vi "test Read Event.vi"(11 "Test Case In":refnum<class "Test PCANBasic.lvclass">) -> (0 "error out":errorcluster, 3 "Test Case Out":refnum<class "Test PCANBasic.lvclass">)   [LabVIEW 2020, in "Test PCANBasic.lvclass"]
uses:
  Test PCANBasic.lvclass
  Test PCANBasic.lvclass/Test PCANBasic.ctl
  C:/Program Files/National Instruments/LabVIEW 2026/vi.lib/Astemes/LUnit/Test Case.lvclass
  C:/Program Files/National Instruments/LabVIEW 2026/vi.lib/Astemes/LUnit/LUnit Runnable.lvclass
  D:/git/PCAN-Basic-LabVIEW/tests/Tests PCANBasic/Test PCANBasic.lvclass
  <vilib>/Astemes/LUnit/Test Case.lvclass
  source/PCANBasic.lvlib
  Global PCAN Channel.vi
  Global PCAN Baudrate.vi
  source/Read Event/Read Event.lvclass
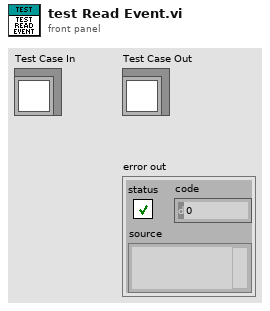
[diagram p1: front panel]
types:
  T1 = cluster{"ID":u32, "MSGTYPE":cluster{"Type":u8, "Extended":bool, "Echo":bool}, "LEN":u8, "DATA":cluster{"0":u8, "1":u8, "2":u8, "3":u8, "4":u8, "5":u8, "6":u8, "7":u8}}
  T2 = typedef "PCANBasic.lvlib/PCAN Baud.ctl" = u16
  T3 = typedef "PCANBasic.lvlib/TPCANHandle.ctl" = u16
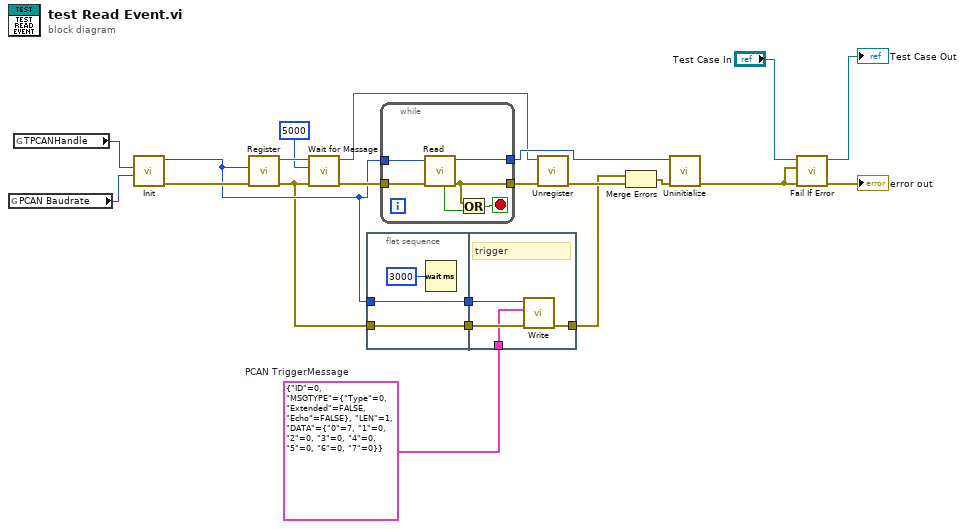
[diagram p0: block diagram]
diagram:
  w1 = T1 {"ID"=0, "MSGTYPE"={"Type"=0, "Extended"=FALSE, "Echo"=FALSE}, "LEN"=1, "DATA"={"0"=7, "1"=0, "2"=0, "3"=0, "4"=0, "5"=0, "6"=0, "7"=0}}  # PCAN TriggerMessage
  n1 = global read "Global PCAN Baudrate.vi" "PCAN Baudrate"() -> (w16:T2)
  n2 = global read "Global PCAN Channel.vi" "TPCANHandle"() -> (w17:T3)
  n3 = call "Init.vi"("Baudrate"=w16, "Channel"=w17) -> ("error out"=w15:errorcluster, "TPCANHandle out"=w10:T3)  [unwired: 7 in, 1 out]
  n4 = call "Register.vi"("error in"=w15, "TPCANHandle"=w10) -> ("error out"=w8:errorcluster, "Read Event out"=w14:refnum<class "Read Event.lvclass">)  [unwired: 8 in]
  n5 = call "Wait for Message.vi"("error in"=w8, "Timeout"=5000, "Read Event in"=w14) -> ("error out"=w12:errorcluster, "Read Event out"=w4:refnum<class "Read Event.lvclass">)  [unwired: 6 in, 1 out]
  n6 = flat-sequence {
    tunnel: w10 -> [w23]
    tunnel: [w23] -> w9
    tunnel: w8 -> [w22]
    tunnel: [w22] -> w7
    tunnel: w9 -> [w28]
    tunnel: w7 -> [w27]
    tunnel: [w26] -> w2
    tunnel: w1 -> [w25]
    frame #0 {
      n7 = Wait (ms)(milliseconds to wait=u32 3000) -> ()  [unwired: 1 out]
    }
    frame #1 {
      # "trigger"
      n8 = call "Write.vi"("error in"=w27, "PCAN Message"=w25, "TPCANHandle in"=w28) -> ("error out"=w26:errorcluster)  [unwired: 6 in, 2 out]
    }
  }
  n9 = while {
    tunnel: w10 -> [w34]
    tunnel: w12 -> [w32]
    tunnel: [w29] -> w11
    tunnel: [w31] -> w6
    stop <- w30 stop-if-true
    n10 = call "Read.vi"("error in"=w32, "TPCANHandle in"=w34) -> ("error out"=w29:errorcluster, "TPCANHandle out"=w31:T3, "Receive Queue empty"=w33:bool)  [unwired: 4 in, 3 out]
    n11 = Or(x=w29, y=w33) -> (x .or. y?=w30:bool)
  }
  n12 = call "Unregister.vi"("error in"=w11, "Read Event in"=w4) -> ("error out"=w5:errorcluster)  [unwired: 8 in, 1 out]
  n13 = Merge Errors(w2, w5) -> (w3:errorcluster)
  n14 = call "Uninitialize.vi"("error in"=w3, "TPCANHandle in"=w6) -> ("error out"=w18:errorcluster)  [unwired: 8 in, 1 out]
  n15 = call <vilib>:"Fail If Error.vi"("error in (no error)"=w18, "Assert error"=w18, "LUnit Test Case In"="Test Case In") -> ("error out"=→"error out":errorcluster, "LUnit Test Case Out"=→"Test Case Out":refnum<class "Test PCANBasic.lvclass">)  [unwired: 7 in]
